vi "startUp.vi"(8 "error in (no error)":errorcluster, 10 "ScriptEvent":refnum<class "ScriptEvent.lvclass">, 11 "playFileAction in":refnum<class "playFileAction.lvclass">) -> (0 "error out":errorcluster, 3 "playFileAction out":refnum<class "playFileAction.lvclass">)   [LabVIEW 2011, in "Views.lvlib" / "ScriptEditor.lvlib" / "playFileAction.lvclass"]
uses:
  playFileAction.lvclass
  Tools/Scripting/ScriptingEvent/ScriptEvent.lvclass
  Tools/Scripting/ScriptingEvent/ScriptEvents/PlayFile/PlayFile.lvclass
  playFileAction.lvclass/playFileAction.ctl
  ActionPanel.lvclass
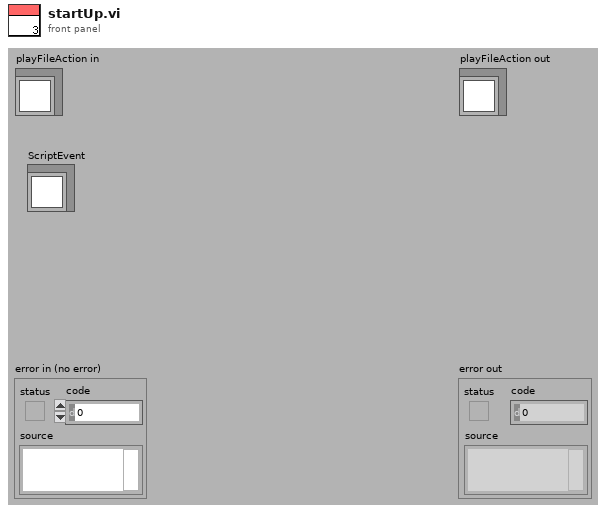
[diagram p1: front panel]
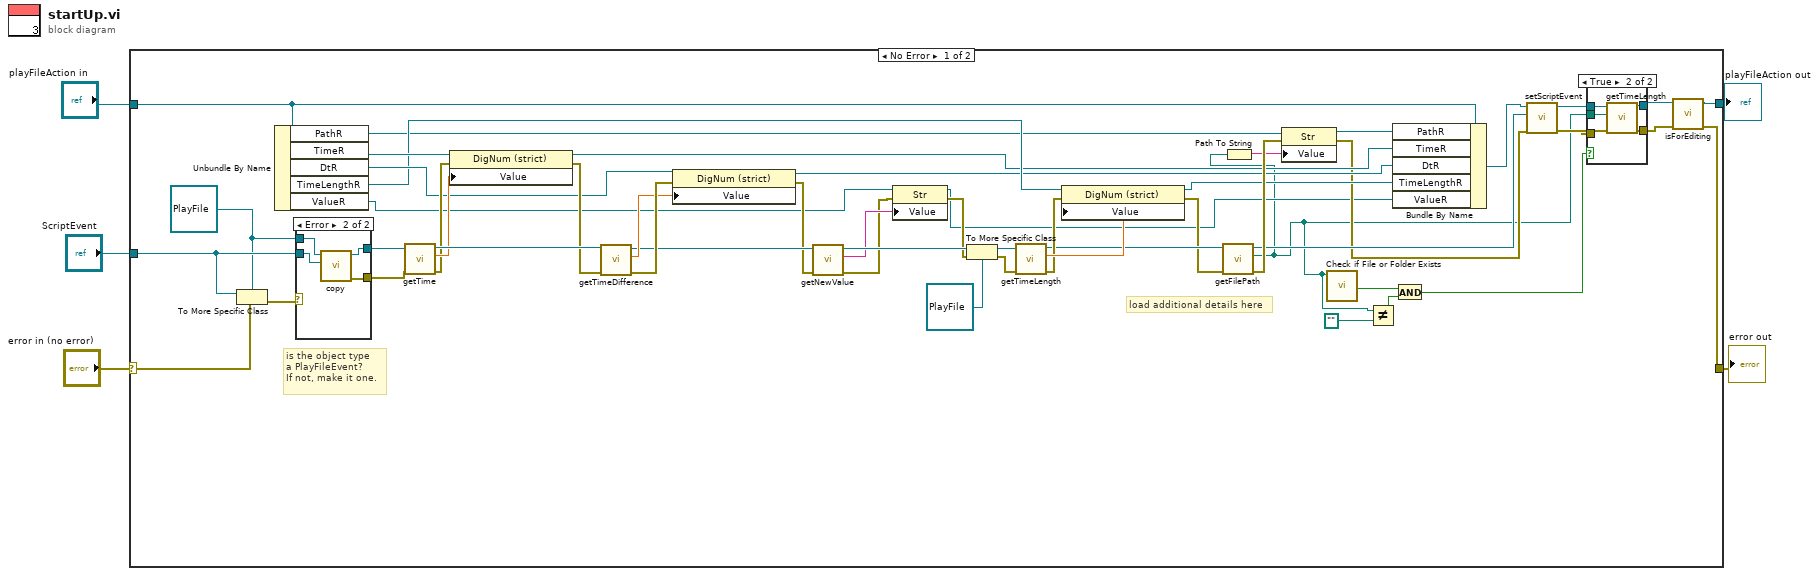
[diagram p0: block diagram]
diagram:
  n1 = case shown="No Error" "error in (no error)" {
    selector: "error in (no error)" -> [w56 w71]
    tunnel: "playFileAction in" -> [w31 w72]
    tunnel: "ScriptEvent" -> [w55 _]
    tunnel: [w53 w72] -> w1
    tunnel: [w54 w71] -> w5
    frame No Error {
      w52 = refnum<class "PlayFile.lvclass"> refnum ("Tools.lvlib:Scripting.lvlib:PlayFile.lvclass")
      # "load additional details here"
      # "is the object type\na PlayFileEvent?\nIf not, make it one."
      n2 = To More Specific Class(target class=w52, reference=w55, error in=w56) -> (error out=w57:errorcluster)  [unwired: 1 out]
      n3 = Unbundle By Name(w31) -> ("PathR"=w33:refnum<vi>, "TimeR"=w47:refnum<vi>, "DtR"=w43:refnum<vi>, "TimeLengthR"=w40:refnum<vi>, "ValueR"=w12:refnum<vi>)
      n4 = case shown="Error" w57 {
        selector: w57 -> [w65 _]
        tunnel: w55 -> [w66 w67]
        tunnel: w52 -> [_ w68]
        tunnel: [w65 w69] -> w49
        tunnel: [w66 w70] -> w48
        frame No Error {
        }
        frame Error {
          n5 = call-dynamic "copy.vi"("ScriptEventForCopy"=w67, "PlayFile in"=w68) -> ("error out"=w69:errorcluster, "PlayFile Copy"=w70:refnum<class "PlayFile.lvclass">)  [unwired: 8 in]
        }
      }
      n6 = call "getTime.vi"("error in (no error)"=w49, "ScriptEvent.lvclass in"=w48) -> ("error out"=w45:errorcluster, "time"=w46:dbl, "ScriptEvent.lvclass out"=w50:refnum<class "ScriptEvent.lvclass">)  [unwired: 7 in]
      n7 = property class="DigNum (strict)"(reference=w47, error in=w45, "Value"=w46) -> (reference out=w29:refnum<vi>, error out=w44:errorcluster)
      n8 = call "getTimeDifference.vi"("error in (no error)"=w44, "ScriptEvent.lvclass in"=w50) -> ("error out"=w42:errorcluster, "time difference"=w41:dbl, "ScriptEvent.lvclass out"=w14:refnum<class "ScriptEvent.lvclass">)  [unwired: 7 in]
      n9 = property class="DigNum (strict)"(reference=w43, error in=w42, "Value"=w41) -> (reference out=w28:refnum<vi>, error out=w13:errorcluster)
      n10 = call "getNewValue.vi"("error in (no error)"=w13, "ScriptEvent.lvclass in"=w14) -> ("error out"=w10:errorcluster, "newValue"=w11:string, "ScriptEvent.lvclass out"=w15:refnum<class "ScriptEvent.lvclass">)  [unwired: 7 in]
      n11 = property class="Str"(reference=w12, error in=w10, "Value"=w11) -> (reference out=w8:refnum<vi>, error out=w9:errorcluster)
      n12 = To More Specific Class(target class=refnum<class "PlayFile.lvclass"> refnum ("Tools.lvlib:Scripting.lvlib:PlayFile.lvclass"), reference=w15, error in=w9) -> (specific class reference=w39:refnum<class "PlayFile.lvclass">, error out=w38:errorcluster)
      n13 = call "getTimeLength.vi"("error in (no error)"=w38, "PlayFile in"=w39) -> ("error out"=w36:errorcluster, "timeLength"=w37:dbl, "PlayFile out"=w35:refnum<class "PlayFile.lvclass">)  [unwired: 7 in]
      n14 = property class="DigNum (strict)"(reference=w40, error in=w36, "Value"=w37) -> (reference out=w27:refnum<vi>, error out=w34:errorcluster)
      n15 = call "getFilePath.vi"("error in (no error)"=w34, "PlayFile in"=w35) -> ("error out"=w32:errorcluster, "filePath"=w6:path, "PlayFile out"=w26:refnum<class "PlayFile.lvclass">)  [unwired: 7 in]
      n16 = Path To String(path=w6) -> (string=w7:string)
      n17 = property class="Str"(reference=w33, error in=w32, "Value"=w7) -> (reference out=w30:refnum<vi>, error out=w25:errorcluster)
      n18 = call <vilib>:"Check if File or Folder Exists.vi"("path"=w6) -> ("file or folder exists?"=w17:bool)  [unwired: 8 in, 2 out]
      n19 = Not Equal?(x=w6, y=path "") -> (x != y?=w19:bool)
      n20 = Bundle By Name(cluster=w31, "PathR"=w30, "TimeR"=w29, "DtR"=w28, "TimeLengthR"=w27, "ValueR"=w8) -> (w24:refnum<class "playFileAction.lvclass">)
      n21 = And(x=w17, y=w19) -> (x .and. y?=w16:bool)
      n22 = call "setScriptEvent.vi"("error in (no error)"=w25, "ScriptEvent.lvclass"=w26, "ActionPanel.lvclass in"=w24) -> ("error out"=w20:errorcluster, "ActionPanel.lvclass out"=w23:refnum<class "playFileAction.lvclass">)  [unwired: 7 in]
      n23 = case shown="True" w16 {
        tunnel: [w59 w64] -> w22
        tunnel: w23 -> [w59 w63]
        tunnel: [w58 w62] -> w21
        tunnel: w20 -> [w58 w61]
        tunnel: w6 -> [_ w60]
        frame False {
        }
        frame True {
          n24 = call "getTimeLength.vi"("error in (no error)"=w61, "Path"=w60, "playFileAction"=w63) -> ("error out"=w62:errorcluster, "playFileAction out"=w64:refnum<class "playFileAction.lvclass">)  [unwired: 6 in, 1 out]
        }
      }
      n25 = call-dynamic "isForEditing.vi"("error in (no error)"=w21, "ActionPanel in"=w22) -> ("error out"=w54:errorcluster, "ActionPanel out"=w53:refnum<class "playFileAction.lvclass">)  [unwired: 7 in, 1 out]
    }
    frame Error {
    }
  }
  "error out" <- w5
  "playFileAction out" <- w1
